vi "Modify IO Pin Names in SPI Engine.vi"(7 "VI to Code Relative Path":string="IONode\\SPIEngineSOM.vi", 8 "Error In":errorcluster, 10 "List of IO Names":string[](array[string])=["Port0/DIO0", "Port0/DIO5"], 11 "Source Root Path":path=path "C:/Users/kvemishe/Downloads/TestScript") -> (0 "Error Out":errorcluster, 1 "Found Object?":bool, 3 "Source Root Path Out":path=path "C:/Users/kvemishe/Downloads/IONode/DLULayer/Dequeue Cmds From Nodes.vi")   [LabVIEW 2014]
doc: "This VI scripts the deque commands VI for the IO Node Engine"
uses:
  <vilib>/Utility/traverseref.llb/TRef TravTarget.ctl
  <vilib>/Utility/traverseref.llb/VI Scripting - Traverse.lvlib
panel:
  out "NumCasesFound":i32
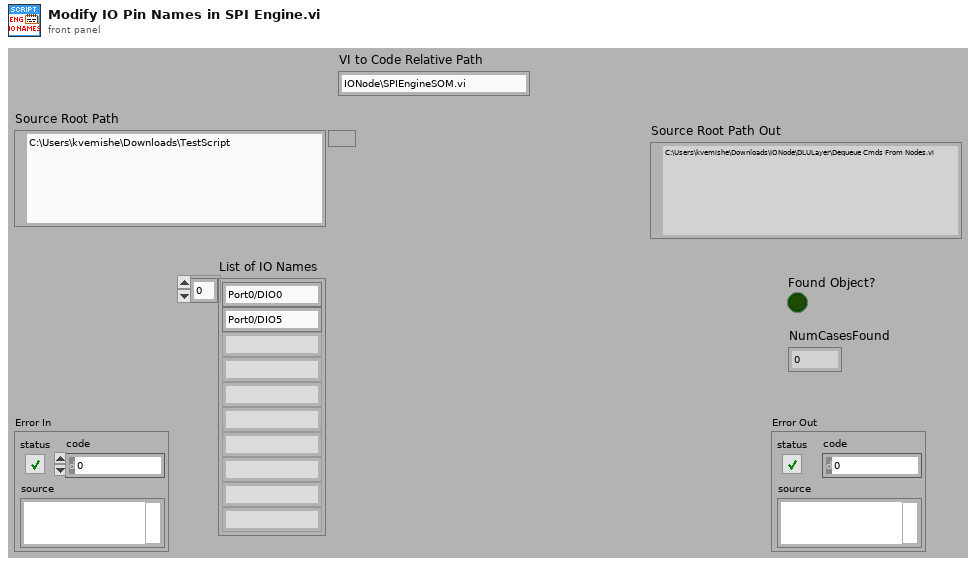
[diagram p1: front panel]
types:
  T1 = typedef "TRef TravTarget.ctl" = enum16{"FP", "BD", "Other"}
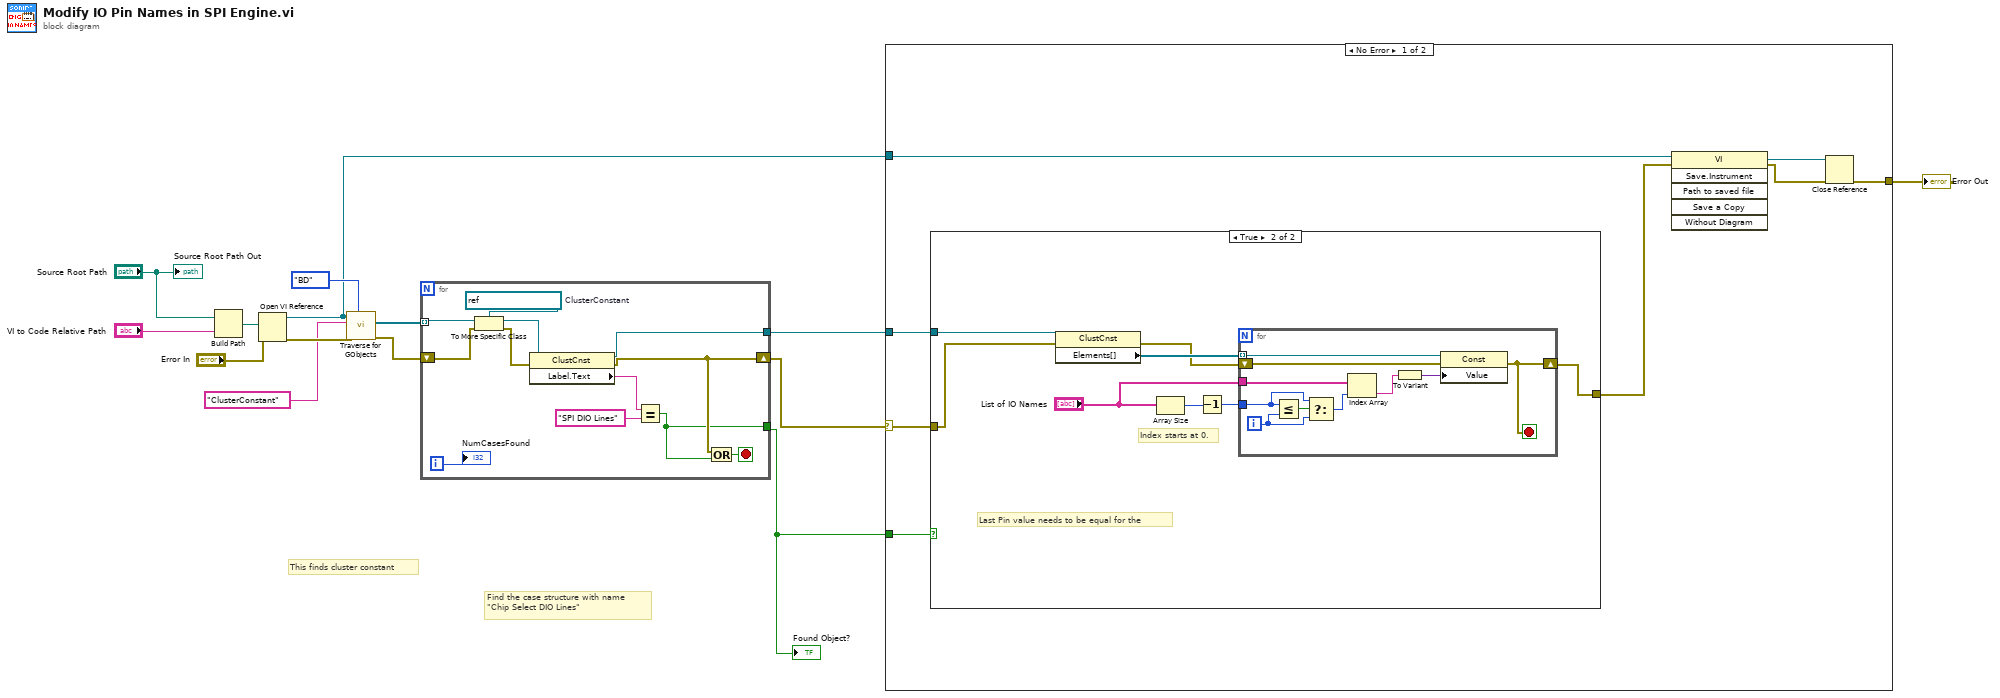
[diagram p0: block diagram]
diagram:
  # "Find the case structure with name\n\"Chip Select DIO Lines\""
  # "This finds cluster constant"
  n1 = Build Path(base path="Source Root Path", name or relative path="VI to Code Relative Path") -> (appended path=w1:path)
  n2 = Open VI Reference(vi path=w1, error in (no error)="Error In") -> (vi reference=w6:refnum<vi>, error out=w13:errorcluster)  [unwired: 4 in]
  n3 = call <vilib>:"Traverse for GObjects.vi"("Traverse Target"=TRef_TravTarget."BD", "error in (no error)"=w13, "Class Name"="ClusterConstant", "VI Refnum"=w6) -> ("error out"=w10:errorcluster, "References"=w11:refnum<vi>[])  [unwired: 4 in, 2 out]
  n4 = for {
    tunnel: w11 -> [w26] mode=indexing
    shift-right: [w18] -> w8
    shift-left: w10 -> [w24]
    tunnel: [w17] -> w7
    tunnel: [w16] -> w9
    i -> [w15]
    stop <- w19 stop-if-true
    w25 = refnum<vi> refnum  # ClusterConstant
    n5 = To More Specific Class(target class=w25, reference=w26, error in=w24) -> (specific class reference=w23:refnum<vi>, error out=w22:errorcluster)
    n6 = property class="ClustCnst"(reference=w23, error in=w22) -> (reference out=w16:refnum<vi>, error out=w18:errorcluster, "Label.Text"=w21:string)
    n7 = Equal?(x=w21, y="SPI DIO Lines") -> (x = y?=w17:bool)
    n8 = Or(x=w18, y=w17) -> (x .or. y?=w19:bool)
    "NumCasesFound" <- w15
  }
  "Found Object?" <- w7
  n9 = case shown="No Error" w8 {
    selector: w8 -> [w32 w54]
    tunnel: w9 -> [w34 _]
    tunnel: w7 -> [w33 _]
    tunnel: w6 -> [w28 _]
    tunnel: [w27 w54] -> w4
    frame No Error {
      n10 = case shown="True" w33 {
        tunnel: w34 -> [_ w41]
        tunnel: w32 -> [w35 w40]
        tunnel: [w35 w39] -> w29
        frame False {
        }
        frame True {
          # "Index starts at 0."
          # "Last Pin value needs to be equal for the"
          n11 = property class="ClustCnst"(reference=w41, error in=w40) -> (error out=w42:errorcluster, "Elements[]"=w43:refnum<vi>[])  [unwired: 1 out]
          n12 = Array Size(array="List of IO Names") -> (size(s)=w37:i32)
          n13 = Decrement(x=w37) -> (x-1=w36:i32)
          n14 = for {
            tunnel: w43 -> [w53] mode=indexing
            tunnel: "List of IO Names" -> [w50]
            shift-right: [w51] -> w39
            shift-left: w42 -> [w52]
            tunnel: w36 -> [w47]
            i -> [w48]
            stop <- w51 stop-if-true
            n15 = Less Or Equal?(x=w47, y=w48) -> (x <= y?=w49:bool)
            n16 = Select(t=w47, s=w49, f=w48) -> (s? t:f=w46:i32)
            n17 = Index Array(array=w50, index=w46) -> (element=w44:string)
            n18 = To Variant(anything=w44) -> (Variant=w45:variant)
            n19 = property class="Const"(reference=w53, error in=w52, "Value"=w45) -> (error out=w51:errorcluster)  [unwired: 1 out]
          }
        }
      }
      n20 = invoke class="VI" method="Save.Instrument"(reference=w28, error in=w29) -> (reference out=w31:refnum<vi>, error out=w30:errorcluster)  [unwired: 4 in, 4 out]
      n21 = Close Reference(reference=w31, error in (no error)=w30) -> (error out=w27:errorcluster)
    }
    frame Error {
    }
  }
  "Error Out" <- w4
  "Source Root Path Out" <- "Source Root Path"
